vi "Line Center Finder.vi"(6 "LineLength":i32, 8 "RadiusIn":i32, 9 "CenterIn":i32, 10 "Line":u8[](array[numeric]), 11 "FirstLine":bool) -> (1 "RadiusOut":i32, 2 "Valid":bool, 3 "CenterOut":i32)   [LabVIEW 2015]
doc: "Scan one line from the center to the sides and looks for the first edge.\nreturns the two edges"
panel:
  out "Line 2":u8[](graph)
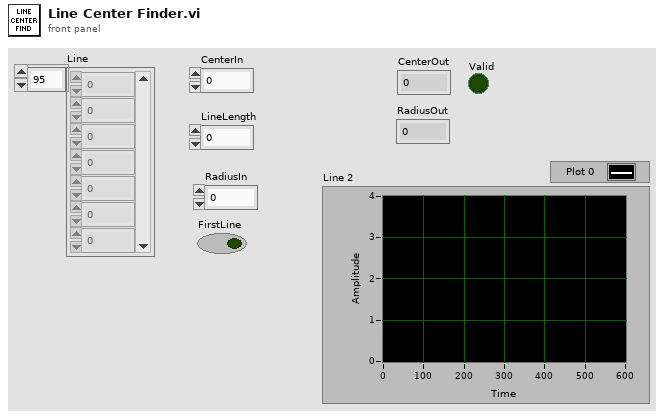
[diagram p1: front panel]
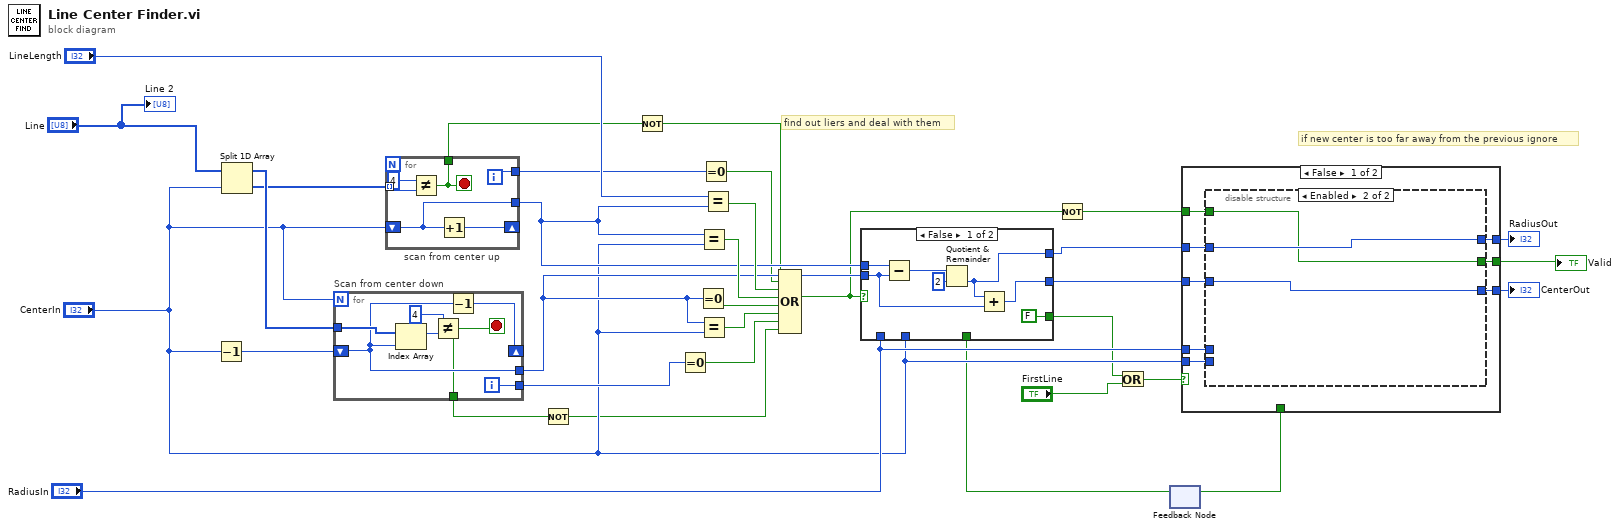
[diagram p0: block diagram]
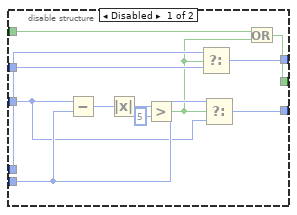
[diagram p2: hidden frame]
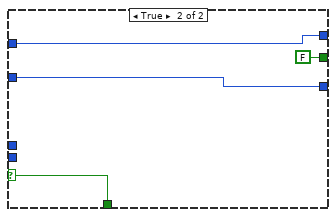
[diagram p3: hidden frame]
diagram:
  # "if new center is too far away from the previous ignore"
  # "find out liers and deal with them"
  n1 = Decrement(x="CenterIn") -> (x-1=w10:i32)
  n2 = Split 1D Array(array="Line", index="CenterIn") -> (first subarray=w32:u8[], second subarray=w31:u8[])
  n3 = for "Scan from center down" {
    N: "CenterIn" -> [_]
    tunnel: w32 -> [w40]
    shift-right: [w39] -> _
    shift-left: w10 -> [w37]
    tunnel: [w37] -> w25
    tunnel: [w35] -> w12
    tunnel: [w34] -> w9
    i -> [w35]
    stop <- w34 stop-if-true
    n4 = Index Array(array=w40, index=w37) -> (element=w38:u8)
    n5 = Not Equal?(x=u8 4, y=w38) -> (x != y?=w34:bool)
    n6 = Decrement(x=w37) -> (x-1=w39:i32)
  }
  n7 = for "scan from center up" {
    tunnel: w31 -> [w46] mode=indexing
    shift-right: [w45] -> _
    shift-left: "CenterIn" -> [w44]
    tunnel: [w44] -> w24
    tunnel: [w42] -> w17
    tunnel: [w41] -> w14
    i -> [w42]
    stop <- w41 stop-if-true
    n8 = Not Equal?(x=u8 4, y=w46) -> (x != y?=w41:bool)
    n9 = Increment(x=w44) -> (x+1=w45:i32)
  }
  n10 = Not(x=w9) -> (.not. x?=w8:bool)
  n11 = Not(x=w14) -> (.not. x?=w13:bool)
  n12 = Equal To 0?(x=w12) -> (x = 0?=w16:bool)
  n13 = Equal To 0?(x=w25) -> (x = 0?=w29:bool)
  n14 = Equal?(x=w24, y="CenterIn") -> (x = y?=w28:bool)
  n15 = Equal?(x=w25, y="CenterIn") -> (x = y?=w30:bool)
  n16 = Equal To 0?(x=w17) -> (x = 0?=w15:bool)
  n17 = Equal?(x="LineLength", y=w24) -> (x = y?=w27:bool)
  n18 = Compound Arithmetic op=OR(w13, w15, w27, w28, w29, w30, w16, w8) -> (w18:bool)
  n19 = Not(x=w18) -> (.not. x?=w1:bool)
  n20 = feedback #1() -> (w7:bool)  [unwired: 1 in]
  n21 = case shown="False" w18 {
    tunnel: [w50 w56] -> w22
    tunnel: w24 -> [w51 _]
    tunnel: w25 -> [w49 _]
    tunnel: "CenterIn" -> [_ w56]
    tunnel: [w48 w55] -> w20
    tunnel: "RadiusIn" -> [_ w55]
    tunnel: w7 -> [_ w54]
    tunnel: [FALSE w54] -> w5
    frame False {
      n22 = Subtract(x=w51, y=w49) -> (x-y=w53:i32)
      n23 = Quotient & Remainder(x=w53, y=2) -> (floor(x/y)=w48:i32)  [unwired: 1 out]
      n24 = Add(x=w48, y=w49) -> (x+y=w50:i32)
    }
    frame True {
    }
  }
  n25 = Or(x=w5, y="FirstLine") -> (x .or. y?=w4:bool)
  n26 = case shown="False" w4 {
    selector: w4 -> [_ w80]
    tunnel: "CenterIn" -> [w64 _]
    tunnel: [w63 w82] -> w23
    tunnel: w22 -> [w62 w82]
    tunnel: "RadiusIn" -> [w61 _]
    tunnel: w20 -> [w60 w83]
    tunnel: [w59 w83] -> w19
    tunnel: [w57 FALSE] -> w2
    tunnel: w1 -> [w58 _]
    tunnel: [_ w80] -> w3
    frame False {
      n27 = disable-structure shown="Enabled" {
        disable-tunnel: w64 -> [w73 _]
        disable-tunnel: [w72 w78] -> w63
        disable-tunnel: w62 -> [w71 w78]
        disable-tunnel: w61 -> [w70 _]
        disable-tunnel: w60 -> [w69 w79]
        disable-tunnel: [w68 w79] -> w59
        disable-tunnel: w58 -> [w66 w77]
        disable-tunnel: [w65 w77] -> w57
        frame Disabled {
          n28 = Subtract(x=w71, y=w73) -> (x-y=w74:i32)
          n29 = Absolute Value(x=w74) -> (abs(x)=w76:i32)
          n30 = Greater?(x=w76, y=5) -> (0:w67:bool)
          n31 = Select(t=w70, s=w67, f=w69) -> (s? t:f=w68:i32)
          n32 = Select(t=w73, s=w67, f=w71) -> (s? t:f=w72:i32)
          n33 = Or(x=w66, y=w67) -> (x .or. y?=w65:bool)
        }
        frame Enabled {
        }
      }
    }
    frame True {
    }
  }
  "CenterOut" <- w23
  "RadiusOut" <- w19
  "Valid" <- w2
  n34 = feedback-in #1(w3) -> ()
  "Line 2" <- "Line"
